vi "Routers.vi"(9 "Controller Map":T1, 10 "Route Handler Map":T3, 11 "Processing In":refnum<class "Processing.lvclass">) -> (0 "error out":errorcluster, 2 "Controller":refnum<class "Controller.lvclass">, 3 "Processing":refnum<class "Processing.lvclass">)   [LabVIEW 2020, in "HTTP Server.lvlib" / "Server.lvclass"]
uses:
  Server.lvclass
  Server.lvclass/Server.ctl
  Processing Step.ctl
  HTTP Server.lvlib
  Processing/Processing.lvclass
  Route Handler/Route Handler.lvclass
  C:/dev/lv20CE/relink/lv-http-server/HTTP Server/Route Handler/Route Handler.lvclass
  C:/dev/lv20CE/relink/lv-http-server/HTTP Server/Handler/Handler.lvclass
  Priority.ctl
  Route Handler Map.ctl
  Controller/Controller.lvclass
  Controller Map.ctl
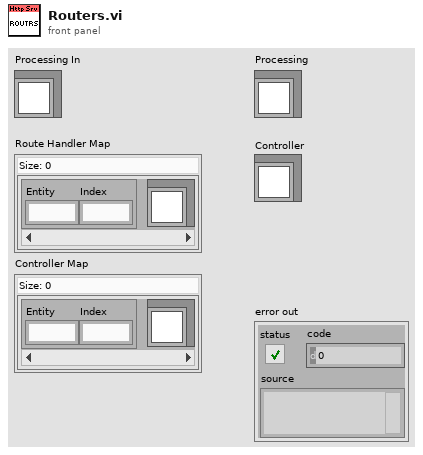
[diagram p1: front panel]
types:
  T1 = typedef "HTTP Server.lvlib/Controller Map.ctl" = map{T2, refnum<class "Controller.lvclass">}
  T2 = typedef "HTTP Server.lvlib/Priority.ctl" = cluster{"Entity":u16, "Index":u16}
  T3 = typedef "HTTP Server.lvlib/Route Handler Map.ctl" = map{T2, refnum<class "Route Handler.lvclass">}
  T4 = typedef "HTTP Server.lvlib/Processing Step.ctl" = enum16{"Connection", "Request", "Routing", "Controller Init", "Controller", "Response", "Complete", "Exception"}
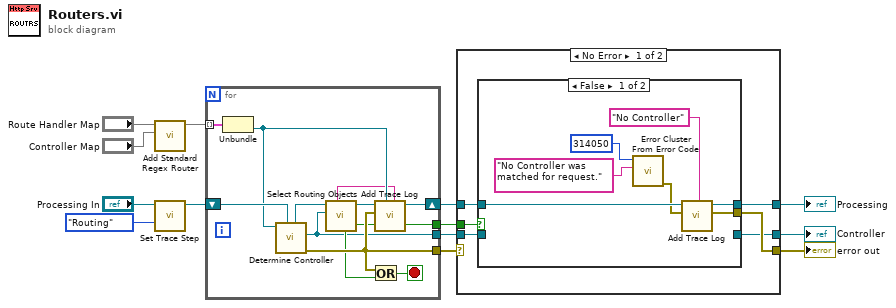
[diagram p0: block diagram]
diagram:
  n1 = call "Add Standard Regex Router.vi"("Controller Map"="Controller Map", "Route Handler Map In"="Route Handler Map") -> ("Route Handler Map"=w10:T3)  [unwired: 9 in]
  n2 = call "Set Trace Step.vi"("Processing Step"=Processing_Step."Routing", "Processing in"="Processing In") -> ("Processing out"=w8:refnum<class "Processing.lvclass">)  [unwired: 9 in]
  n3 = for {
    tunnel: w10 -> [w24] mode=indexing
    shift-right: [w17] -> w5
    shift-left: w8 -> [w22]
    tunnel: [w16] -> w7
    tunnel: [w15] -> w6
    tunnel: [w14] -> w2
    stop <- w23 stop-if-true
    n4 = Unbundle(w24) -> ("Handler"=w19:refnum<class "Route Handler.lvclass">)  [unwired: 1 out]
    n5 = call-dynamic "Determine Controller.vi"("Processing In"=w22, "Route Handler in"=w19) -> ("error out"=w16:errorcluster, "Controller"=w14:refnum<class "Controller.lvclass">, "Processing"=w21:refnum<class "Processing.lvclass">)  [unwired: 7 in]
    n6 = call "Select Routing Objects.vi"("Controller"=w14, "Inputs"=w21) -> ("Updated Inputs"=w20:refnum<class "Processing.lvclass">, "Controller?"=w15:bool, "Trace Message"=w18:string)  [unwired: 7 in]
    n7 = Or(x=w16, y=w15) -> (x .or. y?=w23:bool)
    n8 = call "Add Trace Log.vi"("Info"=w18, "LabVIEW Object"=w19, "error in (no error)"=w16, "Processing in"=w20) -> ("Processing out"=w17:refnum<class "Processing.lvclass">)  [unwired: 6 in, 1 out]
  }
  n9 = case shown="No Error" w7 {
    selector: w7 -> [_ w41]
    tunnel: [w30 w41] -> w13
    tunnel: w6 -> [w29 _]
    tunnel: w5 -> [w28 w40]
    tunnel: [w27 w40] -> w4
    tunnel: w2 -> [w26 _]
    tunnel: [w25 _] -> w1
    frame No Error {
      n10 = case shown="False" w29 {
        tunnel: [w31 _] -> w30
        tunnel: w28 -> [w35 w39]
        tunnel: [w33 w39] -> w27
        tunnel: w26 -> [_ w38]
        tunnel: [_ w38] -> w25
        frame False {
          n11 = call <vilib>:"Error Cluster From Error Code.vi"("error message (\"\")"="No Controller was matched for request." ("error message (\"\")"), "error code (0)"=314050) -> ("error out"=w32:errorcluster)  [unwired: 7 in]
          n12 = call "Add Trace Log.vi"("Info"="No Controller", "error in (no error)"=w32, "Processing in"=w35) -> ("error out"=w31:errorcluster, "Processing out"=w33:refnum<class "Processing.lvclass">)  [unwired: 7 in]
        }
        frame True {
        }
      }
    }
    frame Error {
    }
  }
  "Processing" <- w4
  "error out" <- w13
  "Controller" <- w1
